vi "Choreo_Choreo_LoadAllTrajectories.vi"(8 "error in (no error)":errorcluster) -> (0 "error out":errorcluster, 3 "Trajectories":string[](array[string]))   [LabVIEW 2019, in "ChoreoLib.lvlib"]
doc: "Load all *.traj files found in the default choreo deploy directory into cache. This is an easy way to load everything into memory when the robot is started. All trajectories are expected to be of type Swerve.\n\n\nInputs:\n - ErrorIn - cluster - standard error cluster. Can be used to force execution order.\n\nOutputs:\n - Trajectories - string array - List of the names of the trajectories found and loaded. This is just for information.\n - ErrorOut - cluster - standard error cluster. Can be used to force execution order and check for errors."
uses:
  ChoreoLib.lvlib
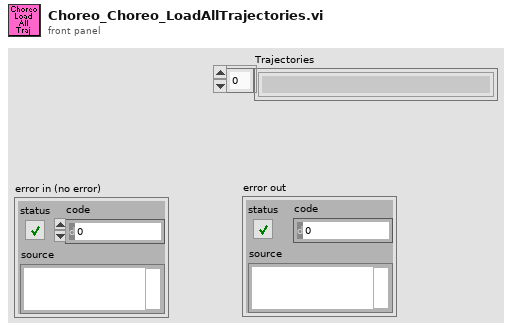
[diagram p1: front panel]
types:
  T1 = typedef "ChoreoLib.lvlib/Choreo_Util_TrajectoryType.ctl" = enum16{"SWERVE", "DIFFERENTIAL", "UNKNOWN"}
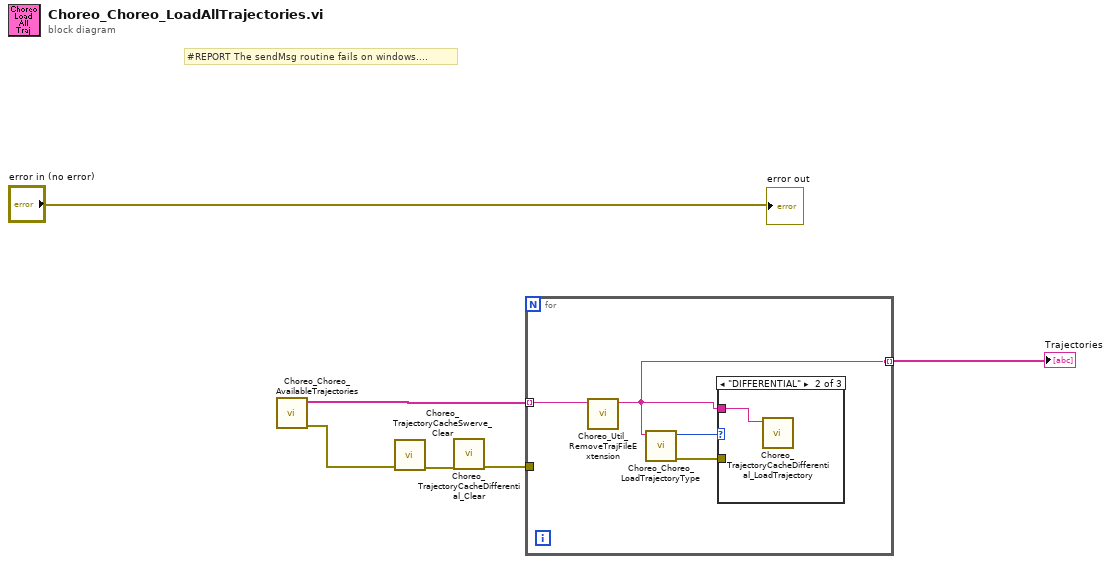
[diagram p0: block diagram]
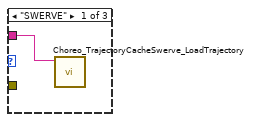
[diagram p2: hidden frame]
diagram:
  # "#REPORT The sendMsg routine fails on windows...."
  n1 = call "Choreo_Choreo_AvailableTrajectories.vi"() -> ("error out"=w3:errorcluster, "filenames"=w6:string[])  [unwired: 9 in, 1 out]
  n2 = call "Choreo_TrajectoryCacheSwerve_Clear.vi"("error in (no error)"=w3) -> ("error out"=w2:errorcluster)  [unwired: 10 in]
  n3 = call "Choreo_TrajectoryCacheDifferential_Clear.vi"("error in (no error)"=w2) -> ("error out"=w1:errorcluster)  [unwired: 10 in]
  n4 = for {
    tunnel: w6 -> [w10] mode=indexing
    tunnel: [w7] -> w5 mode=indexing
    tunnel: w1 -> [_]
    n5 = call "Choreo_Util_RemoveTrajFileExtension.vi"("FileNameIn"=w10) -> ("FileNameOut"=w7:string)  [unwired: 10 in]
    n6 = call "Choreo_Choreo_LoadTrajectoryType.vi"("FileName"=w7) -> ("error out"=w8:errorcluster, "TrajectoryType"=w9:T1)  [unwired: 8 in, 1 out]
    n7 = case shown="\"DIFFERENTIAL\"" w9 {
      tunnel: w8 -> [_ _ _]
      tunnel: w7 -> [w11 w12 _]
      frame "SWERVE" {
        n8 = call "Choreo_TrajectoryCacheSwerve_LoadTrajectory.vi"("TrajectoryName"=w11) -> ()  [unwired: 9 in, 2 out]
      }
      frame "DIFFERENTIAL" {
        n9 = call "Choreo_TrajectoryCacheDifferential_LoadTrajectory.vi"("TrajectoryName"=w12) -> ()  [unwired: 9 in, 2 out]
      }
      frame "UNKNOWN" {
      }
    }
  }
  "Trajectories" <- w5
  "error out" <- "error in (no error)"
